vi "PushLossy.vi"(10 "Element":T1, 11 "POTTypedCircularBuffer in":refnum<class "ErrorLogBuffer.lvclass">) -> (1 "overflow?":bool, 2 "Type":T1, 3 "POTTypedCircularBuffer out":refnum<class "ErrorLogBuffer.lvclass">)   [LabVIEW 2024, in "ErrorLogBuffer.lvclass"]
uses:
  ErrorLogBuffer.lvclass
  Type.ctl
  RQMHCore/ErrorReporting/Record/LogRecord.lvclass
  ErrorLogBuffer.lvclass/ErrorLogBuffer.ctl
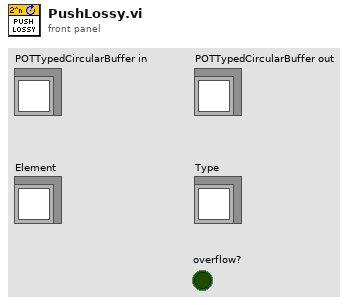
[diagram p1: front panel]
types:
  T1 = typedef "ErrorLogBuffer.lvclass/Type.ctl" = refnum<class "LogRecord.lvclass">
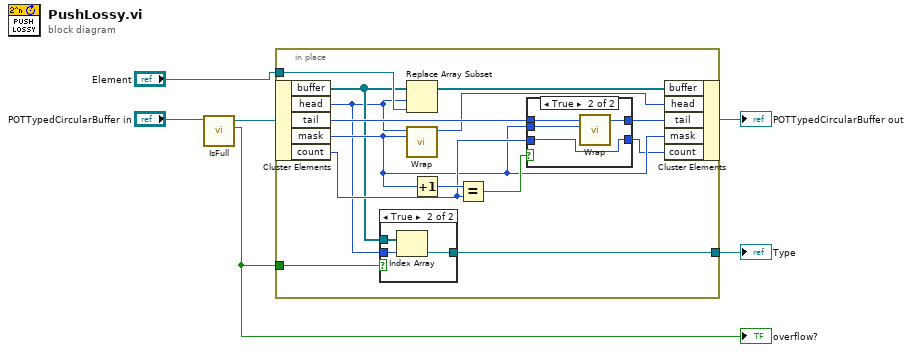
[diagram p0: block diagram]
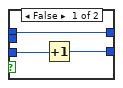
[diagram p3: hidden frame]
diagram:
  n1 = call "IsFull.vi"("POTTypedCircularBuffer in"="POTTypedCircularBuffer in") -> ("Full?"=w1:bool, "POTTypedCircularBuffer out"=w5:refnum<class "ErrorLogBuffer.lvclass">)  [unwired: 9 in]
  "overflow?" <- w1
  n2 = in-place {
    in-place-border: "Element" -> [w19]
    in-place-border: [w8] -> w2
    in-place-border: w1 -> [w7]
    n3 = in-place-cluster #1(w5) -> ("buffer"=w10:T1[], "head"=w9:i32, "tail"=w18:i32, "mask"=w12:i32, "count"=w13:i32)
    n4 = case shown="True" w7 {
      tunnel: w10 -> [_ w23]
      tunnel: w9 -> [_ w22]
      tunnel: [_ w21] -> w8
      frame False {
      }
      frame True {
        n5 = Index Array(array=w23, index=w22) -> (element=w21:T1)
      }
    }
    n6 = Replace Array Subset(array=w10, new element=w19, index=w9) -> (w20:T1[])
    n7 = call "Wrap.vi"("mask"=w12, "index"=w9) -> ("wrapped"=w16:i32)  [unwired: 9 in]
    n8 = Increment(x=w12) -> (x+1=w15:i32)
    n9 = Equal?(x=w15, y=w13) -> (x = y?=w14:bool)
    n10 = case shown="True" w14 {
      tunnel: w18 -> [w26 w30]
      tunnel: w12 -> [_ w29]
      tunnel: [w26 w28] -> w17
      tunnel: w13 -> [w25 w27]
      tunnel: [w24 w27] -> w11
      frame False {
        n11 = Increment(x=w25) -> (x+1=w24:i32)
      }
      frame True {
        n12 = call "Wrap.vi"("mask"=w29, "index"=w30) -> ("wrapped"=w28:i32)  [unwired: 9 in]
      }
    }
    n13 = in-place-cluster #1("buffer"=w20, "head"=w16, "tail"=w17, "mask"=w12, "count"=w11) -> (→"POTTypedCircularBuffer out":refnum<class "ErrorLogBuffer.lvclass">)
  }
  "Type" <- w2
